vi "timeToSeconds.vi"() -> ()   [LabVIEW 2015]
panel:
  out "64bit integer":i64
  out "double precision float":dbl
  out "current time":timestamp
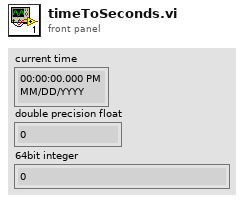
[diagram p1: front panel]
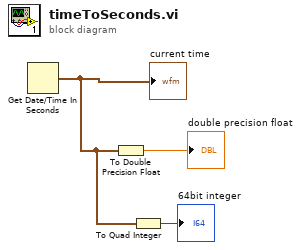
[diagram p0: block diagram]
diagram:
  n1 = Get Date/Time In Seconds() -> (seconds since 1Jan1904=w2:timestamp)
  "current time" <- w2
  n2 = To Double Precision Float(number=w2) -> (double precision float=→"double precision float":dbl)
  n3 = To Quad Integer(1:w2) -> (0:→"64bit integer":i64)
